vi "testDifferentTypes.vi"() -> ()   [LabVIEW 2019, in "AssertionTest.lvlib" / "AssertNotEquals.lvlib"]
uses:
  AssertNotEquals.lvlib
  Assertion/Assertion.lvlib
panel:
  out "error out":errorcluster
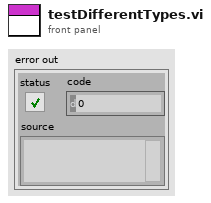
[diagram p1: front panel]
types:
  T1 = cluster{"String":string, "Numeric":i32, "Bool":bool}
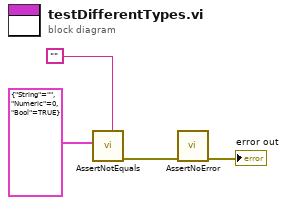
[diagram p0: block diagram]
diagram:
  n1 = call "AssertNotEquals.vi"("Expected"="", "Actual"=T1 {"String"="", "Numeric"=0, "Bool"=TRUE}) -> ("error out"=w2:errorcluster)  [unwired: 9 in]
  n2 = call "AssertNoError.vi"("error in (no error)"=w2) -> ("error out"=→"error out":errorcluster)  [unwired: 10 in]
